vi "dscADScanInt.vi"(8 "error in":errorcluster, 10 "dscAIOint":T1 {"ch_align" items=["FALSE", "TRUE"]; "fifo en" items=["FALSE", "TRUE"]; "int clk gate" items=["FALSE", "TRUE"]; "ext gate en" items=["FALSE", "TRUE"]; "intclk" items=["FALSE", "TRUE"]; "cycle" items=["FALSE", "TRUE"]}, 11 "boardIn":i16) -> (0 "error out":errorcluster, 2 "dscaioint":T1 {"ch_align" items=["FALSE", "TRUE"]; "fifo en" items=["FALSE", "TRUE"]; "int clk gate" items=["FALSE", "TRUE"]; "ext gate en" items=["FALSE", "TRUE"]; "intclk" items=["FALSE", "TRUE"]; "cycle" items=["FALSE", "TRUE"]}, 3 "boardOut":i16)   [LabVIEW 2011, in "Diamond Universal Driver.lvlib"]
doc: "Performs A/D scans using interrupt based IO with one scan per A/D clock tick. Calling this function only starts the interrupt operations in a separate system thread. The function call does not result in an atomic transaction with immediate results. Rather, it starts a real time process that terminates only when the number of conversions reaches the max specified (in one-shot mode) or if a call to <B>dscCancelOp()</B> is made."
uses:
  Diamond Universal Driver.lvlib
  Controls/dscAIOint.ctl
  Controls/dscBool.ctl
  Controls/error codes.ctl
  Instruments/WL OPC/Support/dlls/dscud.dll
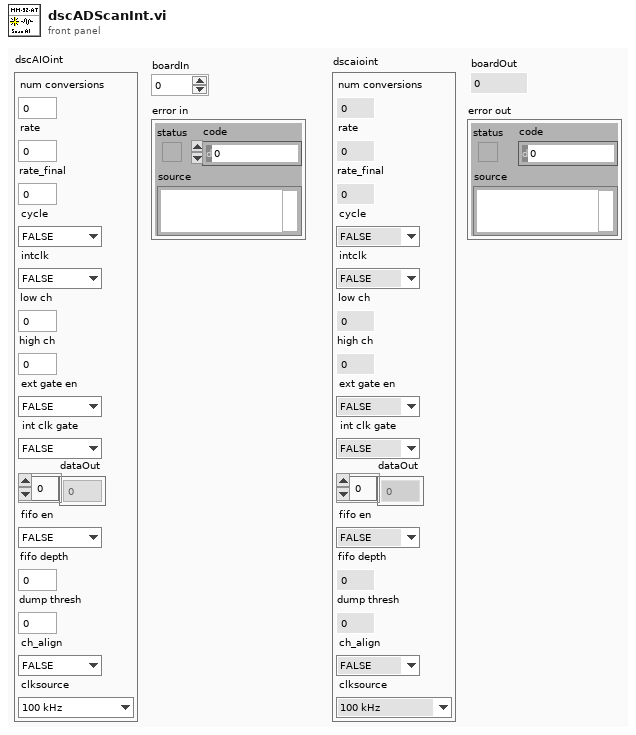
[diagram p1: front panel]
types:
  T1 = typedef "Diamond Universal Driver.lvlib/dscAIOint.ctl" = cluster{"num conversions":u32, "rate":sgl, "rate_final":sgl, "cycle":T2, "intclk":T2, "low ch":u8, "high ch":u8, "ext gate en":T2, "int clk gate":T2, "dataOut":i16[], "fifo en":T2, "fifo depth":u16, "dump thresh":u32, "ch_align":T2, "clksource":enum8{"100 kHz", "1 MHz"}}
  T2 = typedef "dscBool.ctl" = i32
  T3 = typedef "Diamond Universal Driver.lvlib/error codes.ctl" = enum8{"DE_NONE", "DE_HW_FAILURE", "DE_SW_FAILURE", "DE_HW_NOT_SUPPORTED", "DE_SW_NOT_SUPPORTED", "DE_INVALID_PARM", "DE_ALTERNATE_IN_PROGRESS", "DE_NONE_IN_PROGRESS", "DE_BUFFER_ROLLOVER", "DE_INVALID_ERROR_CODE", "DE_ALREADY_PAUSED", "DE_OVERFLOW", "DE_INVALID_FUNC", "DE_DSCUDH_INVALID", "DE_INVALID_BOARD", "DE_BOARD_LIMIT_REACHED", "DE_BOARD_BUSY", "DE_INVALID_WINDRVR_HANDLE", "DE_INVALID_WINDRVR_VERSION", "DE_BAD_WINDRVR_BOARD_INIT", "DE_OPERATION_TIMED_OUT", "DE_INVALID_WINDRVR_KP", "DE_THREAD_FAILURE"}
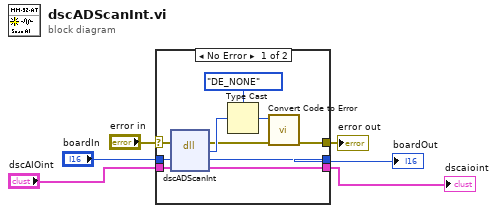
[diagram p0: block diagram]
diagram:
  n1 = case shown="No Error" "error in" {
    selector: "error in" -> [w12 w19]
    tunnel: "dscAIOint" -> [w16 w17]
    tunnel: "boardIn" -> [w15 w18]
    tunnel: [w14 w17] -> w4
    tunnel: [w13 w18] -> w3
    tunnel: [w7 w19] -> w1
    frame No Error {
      n2 = dll-call lib="C:/Users/mrichardson/Documents/Web Based Version Control SW/Instruments/WL OPC/Support/dlls/dscud.dll" fn="dscADScanInt"(error in=w12, "board"=w15, "dscaioint"=w16) -> (error out=w9:errorcluster, "error"=w10:u8, "board"=w13:i16, "dscaioint"=w14:T1)  [unwired: 2 in, 1 out]
      n3 = Type Cast(type=error_codes."DE_NONE" ("error codes"), x=w10) -> (*(type *) &x=w8:T3)
      n4 = call "Convert Code to Error.vi"("error in"=w9, "error codes"=w8) -> ("error out"=w7:errorcluster)  [unwired: 9 in]
    }
    frame Error {
    }
  }
  "dscaioint" <- w4
  "boardOut" <- w3
  "error out" <- w1
